vi "write_data.vi"(8 "error in (no error)":errorcluster, 10 "data":T1, 11 "MultiTaskLasso in":refnum<class "MultiTaskLasso.lvclass">) -> (0 "error out":errorcluster, 3 "MultiTaskLasso out":refnum<class "MultiTaskLasso.lvclass">)   [LabVIEW 2020, in "MultiTaskLasso.lvclass"]
uses:
  MultiTaskLasso.lvclass
  Controls/multi_task_lasso_data.ctl
  MultiTaskLasso.lvclass/MultiTaskLasso.ctl
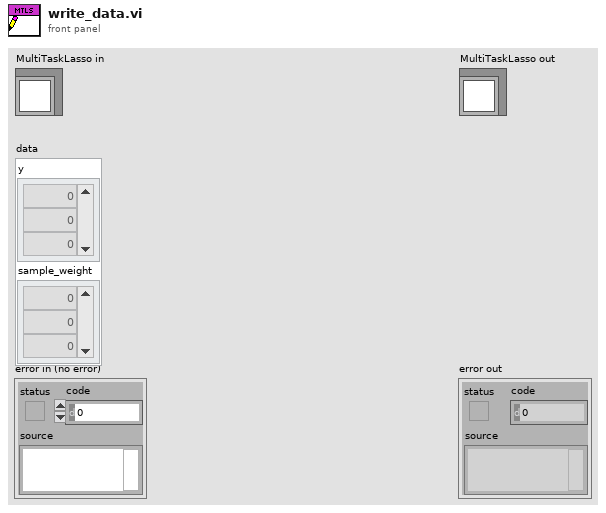
[diagram p1: front panel]
types:
  T1 = typedef "multi_task_lasso_data.ctl" = cluster{"y":dbl[][], "sample_weight":dbl[]}
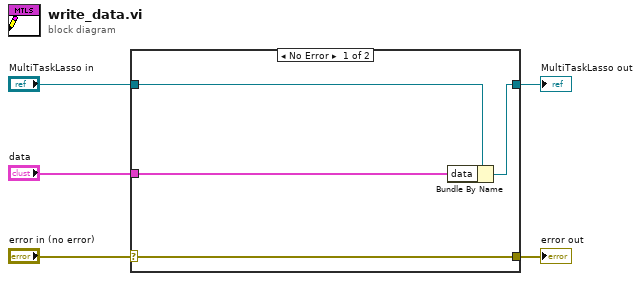
[diagram p0: block diagram]
diagram:
  n1 = case shown="No Error" "error in (no error)" {
    selector: "error in (no error)" -> [w9 w10]
    tunnel: [w9 w10] -> w4
    tunnel: [w7 w11] -> w2
    tunnel: "MultiTaskLasso in" -> [w8 w11]
    tunnel: "data" -> [w6 _]
    frame No Error {
      n2 = Bundle By Name(cluster=w8, "data"=w6) -> (w7:refnum<class "MultiTaskLasso.lvclass">)
    }
    frame Error {
    }
  }
  "error out" <- w4
  "MultiTaskLasso out" <- w2
